vi "Ping.vi"(11 "IP Address":string="127.0.0.1") -> (3 "Available?":bool)   [LabVIEW 2019]
panel:
  out "Status":i32(ring) items=["Success"=0, "DestinationNetworkUnreachable"=11002, "DestinationHostUnreachable"=11003, "DestinationProhibited, DestinationProtocolUnreachable"=11004, "DestinationPortUnreachable"=11005, "NoResources"=11006, "BadOption"=11007, "HardwareError"=11008, "PacketTooBig"=11009, "TimedOut"=11010, "BadRoute"=11012, "TtlExpired"=11013, "TtlReassemblyTimeExceeded"=11014, "ParameterProblem"=11015, "SourceQuench"=11016, "BadDestination"=11018, "DestinationUnreachable"=11040, "TimeExceeded"=11041, "BadHeader"=11042, "UnrecognizedNextHeader"=11043, "IcmpError"=11044, "DestinationScopeMismatch"=11045, "Unknown"=-1]
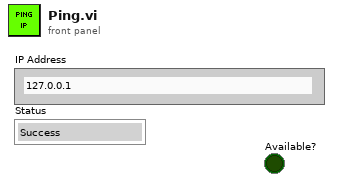
[diagram p1: front panel]
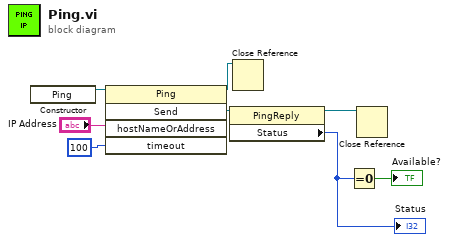
[diagram p0: block diagram]
diagram:
  n1 = constructor class="Ping"() -> (reference out=w5:refnum<k24>)  [unwired: 3 in, 2 out]
  n2 = invoke class="Ping" method="Send"(reference=w5, "hostNameOrAddress"="IP Address", "timeout"=100) -> (reference out=w3:refnum<k24>, "Send"=w7:refnum<k24>)  [unwired: 2 in, 3 out]
  n3 = property class="PingReply"(reference=w7) -> (reference out=w4:refnum<k24>, "Status"=w1:i32)  [unwired: 1 in, 1 out]
  "Status" <- w1
  n4 = Close Reference(reference=w3) -> ()  [unwired: 1 in, 1 out]
  n5 = Equal To 0?(x=w1) -> (x = 0?=→"Available?":bool)
  n6 = Close Reference(reference=w4) -> ()  [unwired: 1 in, 1 out]
